vi "S2DS_config_loading_instruction.vi"(11 "Loading information in":bool[](array[boolean])) -> (3 "Loading information out":bool[](array[boolean]))   [LabVIEW 2025]
panel:
  in  "Common info":bool
  in  "Select None":bool
  in  "Select all":bool
  in  "OK":bool
  in  "Data analysis info":bool
  in  "Read channel info":bool
  in  "Write channel info (!)":bool
  in  "Sweep info":bool=TRUE
  # "SELECT WHAT TO LOAD"
  # "(!) Does not update present value or the target. \nUpdates rest of the stuffs, i.e., factors, step, bin, rate."
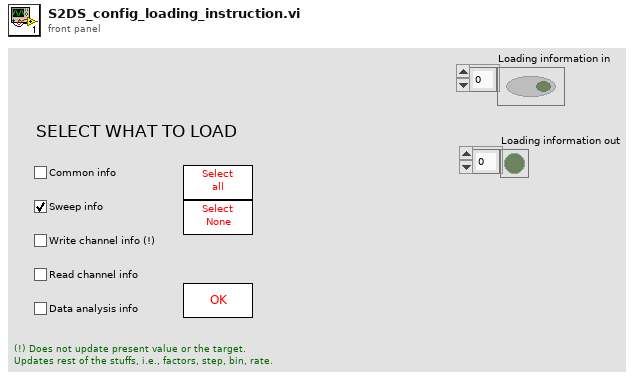
[diagram p1: front panel]
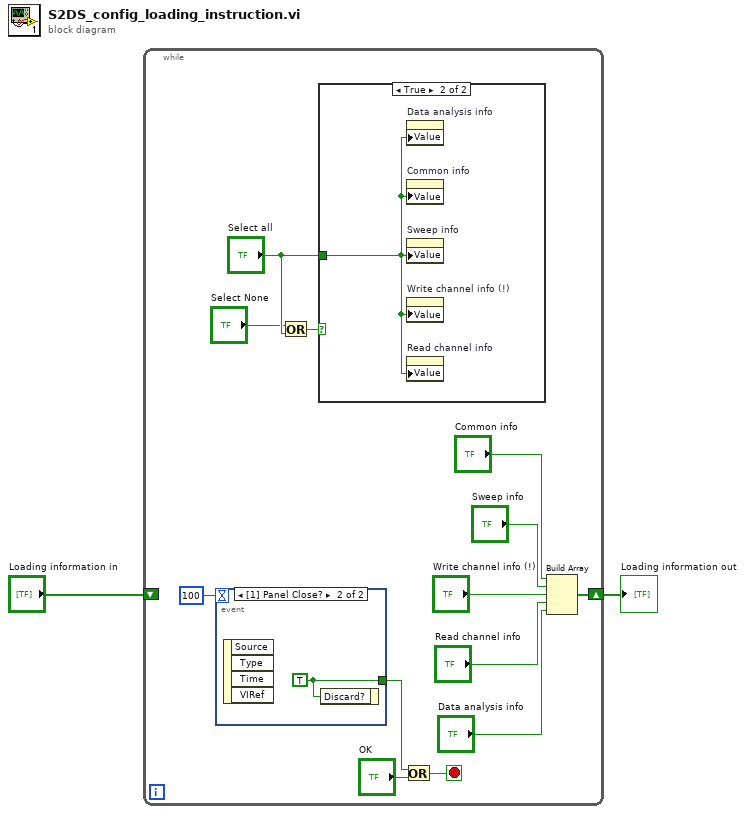
[diagram p0: block diagram]
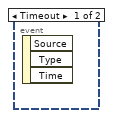
[diagram p3: hidden frame]
diagram:
  n1 = while {
    shift-right: [w8] -> w2
    shift-left: "Loading information in" -> [_]
    stop <- w9 stop-if-true
    n2 = event shown="[1] Panel Close?" {
      selector: _ -> [_ _]
      dyn-events: _ -> [_ _]
      timeout: 100 -> [_ _]
      tunnel: [_ w17] -> w11
      event Timeout {
        n3 = event-data() -> ()  [unwired: 1 in, 3 out]
      }
      event Panel Close? {
        w17 = TRUE ("Discard?")
        n4 = event-data() -> ()  [unwired: 1 in, 4 out]
        n5 = event-data("Discard?"=w17) -> ()  [unwired: 1 in, 1 out]
      }
    }
    n6 = Or(x="Select None", y="Select all") -> (x .or. y?=w4:bool)
    n7 = case shown="True" w4 {
      tunnel: "Select all" -> [_ w16]
      frame False {
      }
      frame True {
        n8 = property on="Data analysis info" class="Bool (strict)"("Value"=w16) -> ()  [unwired: 2 in, 2 out]
        n9 = property on="Common info" class="Bool (strict)"("Value"=w16) -> ()  [unwired: 2 in, 2 out]
        n10 = property on="Sweep info" class="Bool (strict)"("Value"=w16) -> ()  [unwired: 2 in, 2 out]
        n11 = property on="Write channel info (!)" class="Bool (strict)"("Value"=w16) -> ()  [unwired: 2 in, 2 out]
        n12 = property on="Read channel info" class="Bool (strict)"("Value"=w16) -> ()  [unwired: 2 in, 2 out]
      }
    }
    n13 = Or(x=w11, y="OK") -> (x .or. y?=w9:bool)
    n14 = Build Array("Common info", "Sweep info", "Write channel info (!)", "Read channel info", "Data analysis info") -> (w8:bool[])
  }
  "Loading information out" <- w2
